vi "Inject Attribute List.vi"(6 "Attributes Ref":refnum<data-value>, 8 "error in (no error)":errorcluster, 11 "Start Pre-Soak in":refnum<class "Wait.lvclass">) -> (0 "error out":errorcluster, 3 "Start Pre-Soak out":refnum<class "Wait.lvclass">)   [LabVIEW 2019, in "Wait.lvclass"]
uses:
  <vilib>/gpm_packages/@cs/Car-wash/Source/Process Steps/Wait/Wait.lvclass
  <vilib>/gpm_packages/@cs/lookup-table/Source/LookupTable/LookupTable.lvclass
  <vilib>/gpm_packages/@cs/lookup-table/Source/LookupTable/LookupTable.lvclass/LookupTable.ctl
  <vilib>/gpm_packages/@cs/Car-wash/Source/Process Steps/Wait/Wait.lvclass/Wait.ctl
  a44463a7-0659-4e4d-b82a-4fa02a3b5f38.vi
  <vilib>/gpm_packages/@cs/lookup-table/Source/LookupTable/Read Table Reference.vi
  a44463a7-0659-4e4d-b82a-4fa02a3b5f38.vi/6b83685e-9d14-4956-877c-fe10fce445dd.vi
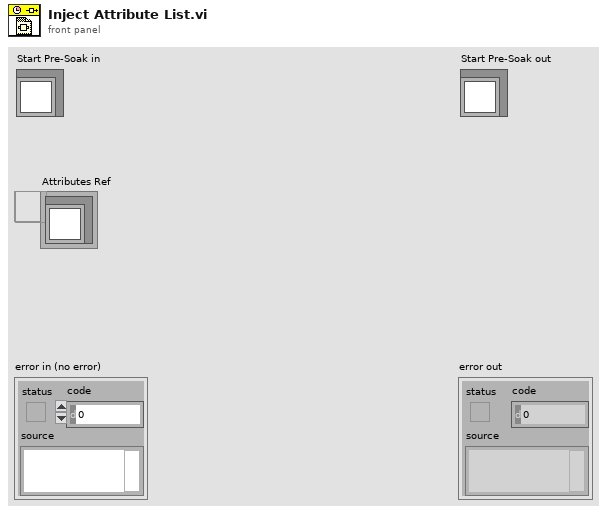
[diagram p1: front panel]
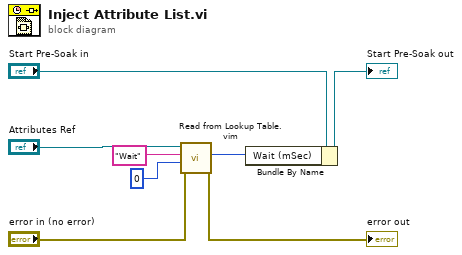
[diagram p0: block diagram]
diagram:
  n1 = call "Read from Lookup Table.vim"("error in (no error)"="error in (no error)", "Type"=0, "Item Name"="Wait", "LookupTable Reference"="Attributes Ref") -> ("error out"=→"error out":errorcluster, "Value"=w3:i32)  [unwired: 4 in, 2 out]
  n2 = Bundle By Name(cluster="Start Pre-Soak in", "Wait (mSec)"=w3) -> (→"Start Pre-Soak out":refnum<class "Wait.lvclass">)
